vi "WriteVirtualSetup.vi"(8 "error in (no error)":errorcluster, 10 "AllVirtualTypeData":T1={"Search Name"="", "Start X"=0.0, "Increase X"=0.0, "X Step"=1, "Start Y"=0.0, "Increase Y"=0.0, "Y Step"=1, "Sensor"=0} {"Y Step" min=1 step=1; "X Step" min=1 step=1}, 11 "Project.lvclass In":refnum<class "Project.lvclass">) -> (0 "error out":errorcluster, 3 "Project.lvclass Out":refnum<class "Project.lvclass">)   [LabVIEW 2014, in "Project.lvclass"]
uses:
  Project.lvclass
  Virtual/Control/AllVirtualTypeData.ctl
  Project.lvclass/Project.ctl
  Virtual/VirtualOrigin.lvclass
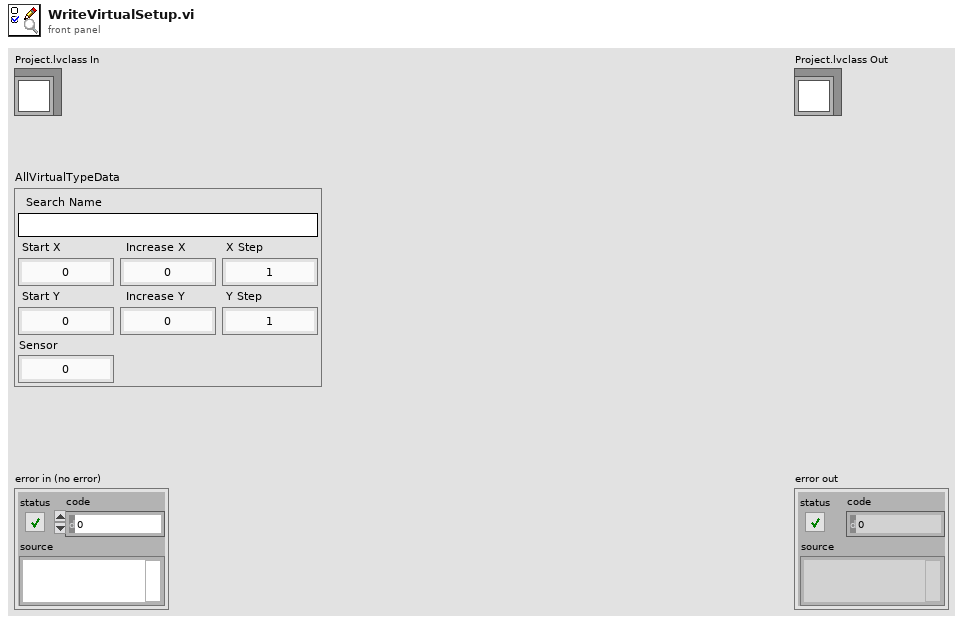
[diagram p1: front panel]
types:
  T1 = typedef "VirtualOrigin.lvclass/AllVirtualTypeData.ctl" = cluster{"Search Name":string, "Start X":dbl, "Increase X":dbl, "X Step":i32, "Start Y":dbl, "Increase Y":dbl, "Y Step":i32, "Sensor":i32}
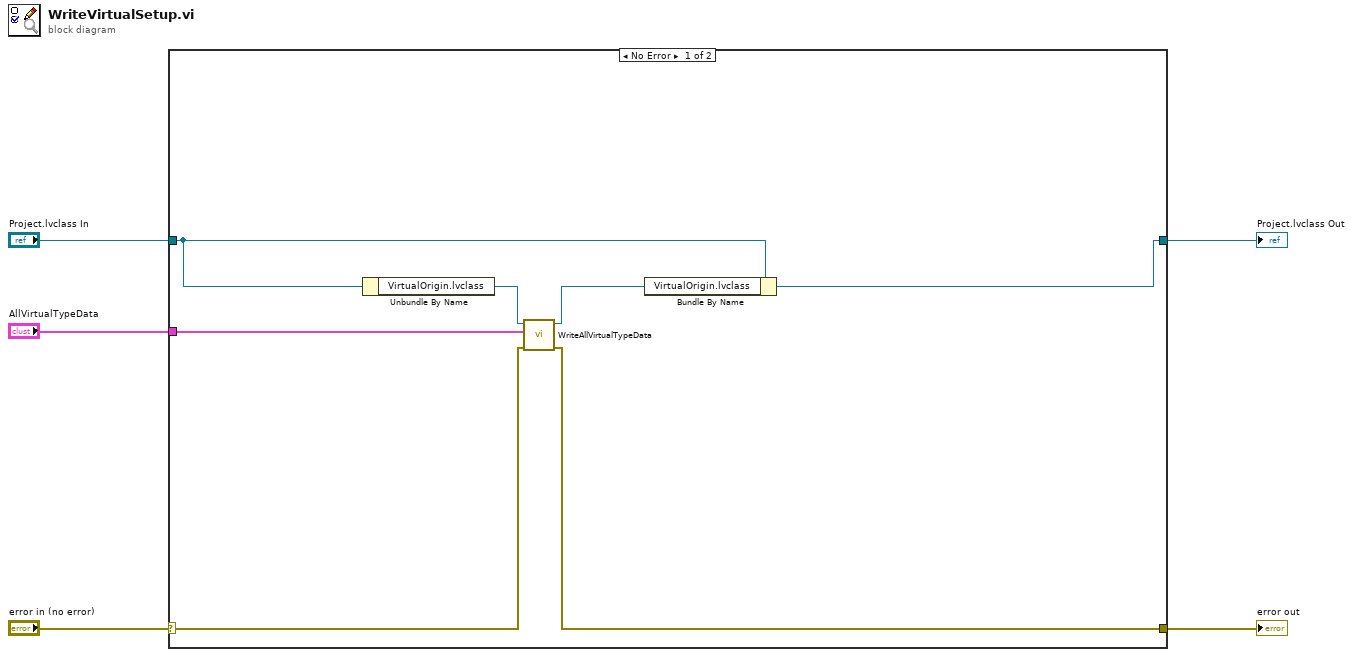
[diagram p0: block diagram]
diagram:
  n1 = case shown="No Error" "error in (no error)" {
    selector: "error in (no error)" -> [w10 w14]
    tunnel: [w9 w14] -> w4
    tunnel: "Project.lvclass In" -> [w7 w13]
    tunnel: [w12 w13] -> w2
    tunnel: "AllVirtualTypeData" -> [w6 _]
    frame No Error {
      n2 = Unbundle By Name(w7) -> ("VirtualOrigin.lvclass"=w8:refnum<class "VirtualOrigin.lvclass">)
      n3 = call "WriteAllVirtualTypeData.vi"("error in (no error)"=w10, "AllVirtualTypeData In"=w6, "VirtualOrigin.lvclass In"=w8) -> ("error out"=w9:errorcluster, "VirtualOrigin.lvclass Out"=w11:refnum<class "VirtualOrigin.lvclass">)  [unwired: 7 in]
      n4 = Bundle By Name(cluster=w7, "VirtualOrigin.lvclass"=w11) -> (w12:refnum<class "Project.lvclass">)
    }
    frame Error {
    }
  }
  "error out" <- w4
  "Project.lvclass Out" <- w2
